vi "JSON Parse Info.vi"(0 "JSON":string, 11 "error in (no error)":errorcluster) -> (4 "results-JSON":string caption="results-JSON string", 6 "ID":i32, 15 "error out":errorcluster)   [LabVIEW 2023, in "Communicator.lvclass"]
doc: "Wrapper around all other VIs that parse an answer from the ICL."
uses:
  Communicator.lvclass
panel:
  # "Connector Pane"
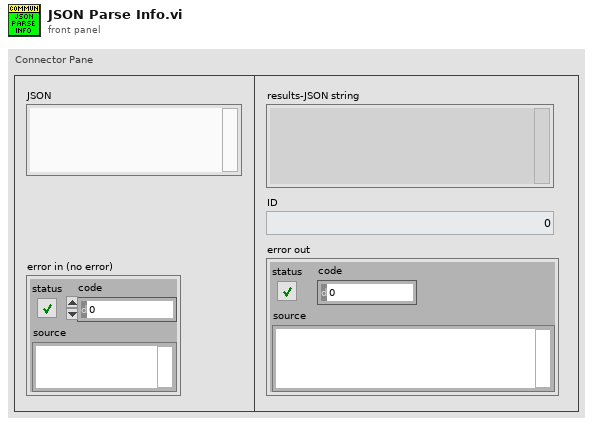
[diagram p1: front panel]
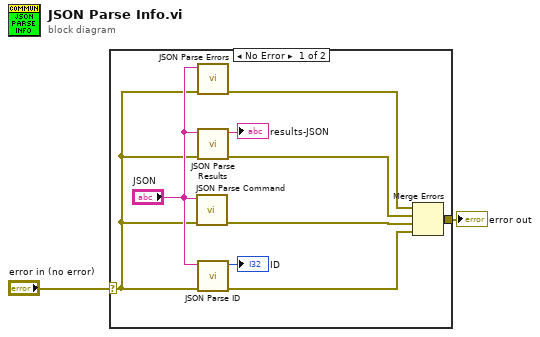
[diagram p0: block diagram]
diagram:
  n1 = case shown="No Error" "error in (no error)" {
    selector: "error in (no error)" -> [w3 w12]
    tunnel: [w10 w12] -> w2
    frame No Error {
      n2 = call "JSON Parse Command.vi"("error in (no error)"=w3, "JSON command"="JSON") -> ("error out"=w5:errorcluster)  [unwired: 7 in, 2 out]
      n3 = call "JSON Parse Errors.vi"("error in (no error)"=w3, "JSON command"="JSON") -> ("error out"=w7:errorcluster)  [unwired: 7 in, 2 out]
      n4 = call "JSON Parse Results.vi"("error in (no error)"=w3, "JSON"="JSON") -> ("error out"=w6:errorcluster, "results-JSON"=→"results-JSON":string)  [unwired: 7 in, 1 out]
      n5 = call "JSON Parse ID.vi"("error in (no error)"=w3, "JSON"="JSON") -> ("error out"=w4:errorcluster, "ID"=→"ID":i32)  [unwired: 7 in, 1 out]
      n6 = Merge Errors(w7, w6, w5, w4) -> (w10:errorcluster)
    }
    frame Error {
    }
  }
  "error out" <- w2
